vi "OP500ZP_SCANequipements.vi"(8 "Errin":errorcluster caption="errin", 10 "Chaîne":string="Log et conf\\Config.ini", 11 "pathin":path=path "D:/CODE/02 SLIM ZEN") -> (0 "ERROUT":errorcluster caption="error out", 1 "KO?":bool=TRUE, 3 "VISA OUT":T1)   [LabVIEW 2020]
doc: "Ce vi il détecte la presence des équipements"
uses:
  VG/VG_ATEQ.vi
  VG/VG_ST5520.vi
  VG/VG_BT3562.vi
  VG/VG_MX5060.vi
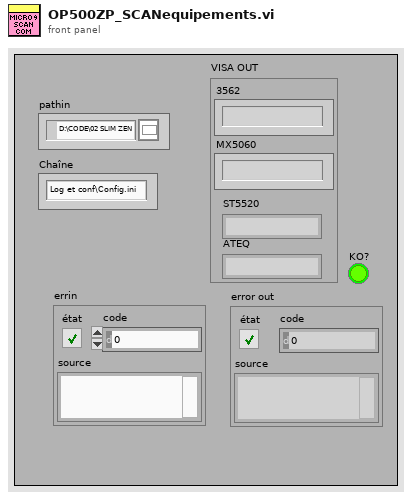
[diagram p1: front panel]
types:
  T1 = cluster{"3562":string, "MX5060":string, "ST5520":string, "ATEQ":string}
  T2 = cluster{"3564":string, "MX5060":string, "ST5520":string, "ATEQ":string}
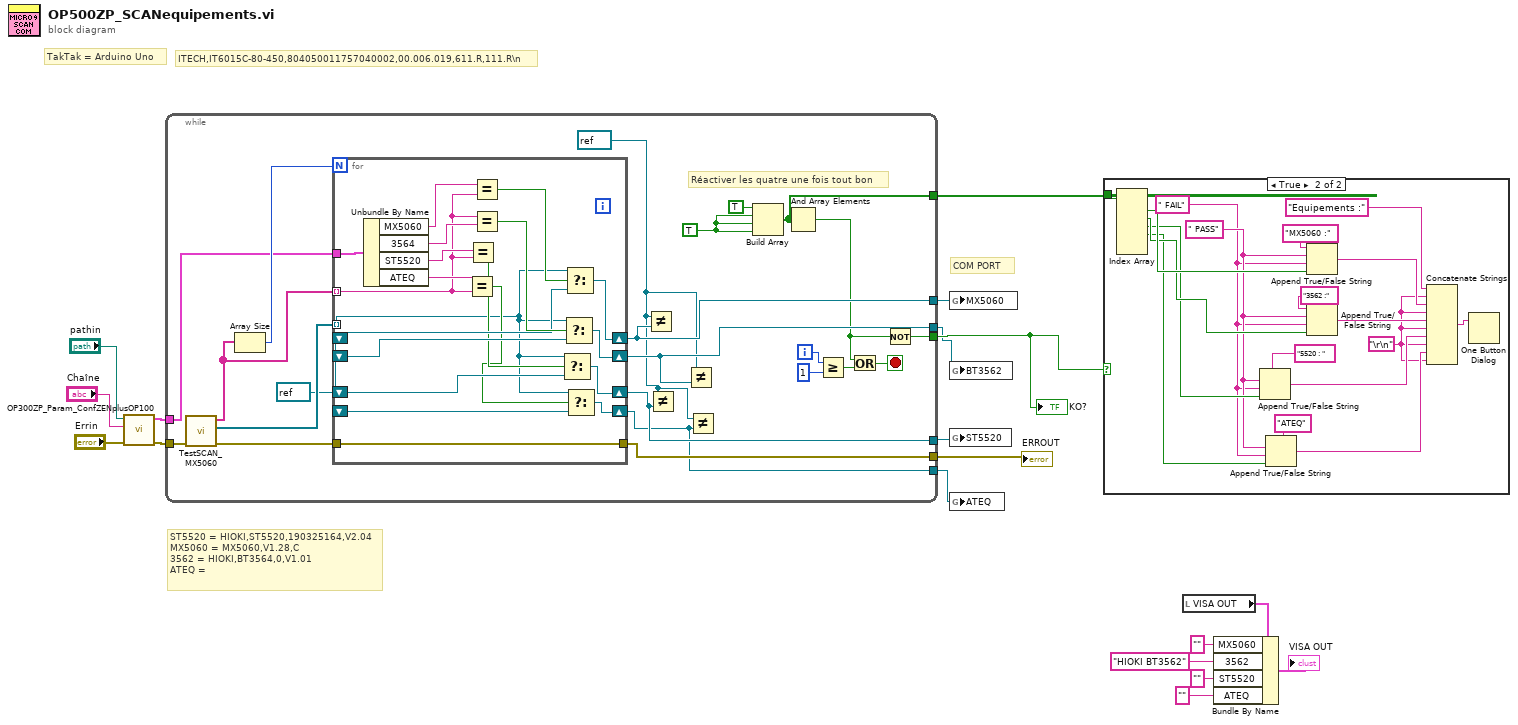
[diagram p0: block diagram]
diagram:
  # "ST5520 = HIOKI,ST5520,190325164,V2.04\t\nMX5060 = MX5060,V1.28,C\n3562 = HIOKI,BT3564,0,V1.01\nATEQ ="
  # "COM PORT"
  # "TakTak = Arduino Uno"
  # "ITECH,IT6015C-80-450,804050011757040002,00.006.019,611.R,111.R\\n"
  n1 = call "OP300ZP_Param_ConfZENplusOP100.vi"("errin"="Errin", "Chaîne"="Chaîne", "pathin"="pathin") -> ("errout"=w15:errorcluster, "VISA OUT"=w14:T2)  [unwired: 7 in]
  n2 = while {
    tunnel: [w30] -> w6
    tunnel: [w29] -> w7
    tunnel: w15 -> [w39]
    tunnel: [w34] -> w18
    tunnel: w14 -> [w31]
    tunnel: [w27] -> w17
    tunnel: [w25] -> w5
    tunnel: [w23] -> w1
    tunnel: [w21] -> w4
    i -> [w33]
    stop <- w36 stop-if-true
    w19 = TRUE ("élément")
    w22 = refnum<visa-resource-name> refnum ("x")
    w26 = refnum<visa-resource-name> refnum ("VISA resource name out")
    # "Réactiver les quatre une fois tout bon"
    n3 = call "TestSCAN_MX5060.vi"("errin"=w39) -> ("error out"=w24:errorcluster, "Tableau 2"=w37:refnum<visa-resource-name>[], "Tableau"=w38:string[])  [unwired: 8 in]
    n4 = Array Size(array=w38) -> (size(s)=w40:i32)
    n5 = for {
      N: w40 -> [_]
      shift-right: [w58] -> w30
      shift-left: w26 -> [w56]
      shift-right: [w57] -> w29
      shift-left: w26 -> [w55]
      tunnel: w38 -> [w45] mode=indexing
      tunnel: w31 -> [w54]
      shift-right: [w51] -> w25
      shift-left: w26 -> [w52]
      tunnel: w37 -> [w43] mode=indexing
      tunnel: w24 -> [w47]
      tunnel: [w47] -> w23
      shift-right: [w42] -> w21
      shift-left: _ -> [w41]
      n6 = Unbundle By Name(w54) -> ("MX5060"=w53:string, "3564"=w48:string, "ST5520"=w50:string, "ATEQ"=w46:string)
      n7 = Equal?(x=w46, y=w45) -> (x = y?=w44:bool)
      n8 = Equal?(x=w50, y=w45) -> (x = y?=w49:bool)
      n9 = Equal?(x=w53, y=w45) -> (x = y?=w59:bool)
      n10 = Equal?(x=w45, y=w48) -> (x = y?=w60:bool)
      n11 = Select(t=w43, s=w49, f=w52) -> (s? t:f=w51:refnum<visa-resource-name>)
      n12 = Select(t=w43, s=w60, f=w55) -> (s? t:f=w57:refnum<visa-resource-name>)
      n13 = Select(t=w43, s=w59, f=w56) -> (s? t:f=w58:refnum<visa-resource-name>)
      n14 = Select(t=w43, s=w44, f=w41) -> (s? t:f=w42:refnum<visa-resource-name>)
    }
    n15 = Not Equal?(x=w22, y=w30) -> ()  [unwired: 1 out]
    n16 = Not Equal?(x=w22, y=w25) -> ()  [unwired: 1 out]
    n17 = Not Equal?(x=w22, y=w29) -> ()  [unwired: 1 out]
    n18 = Not Equal?(x=w22, y=w21) -> ()  [unwired: 1 out]
    n19 = Build Array(TRUE ("élément"), w19, w19, w19) -> (w27:bool[])
    n20 = And Array Elements(Boolean array=w27) -> (logical AND=w28:bool)
    n21 = Greater Or Equal?(x=w33, y=1) -> (x >= y?=w35:bool)
    n22 = Or(x=w28, y=w35) -> (x .or. y?=w36:bool)
    n23 = Not(x=w28) -> (.not. x?=w34:bool)
  }
  "KO?" <- w18
  "ERROUT" <- w1
  n24 = global write "VG_MX5060.vi" "MX5060"(w6) -> ()
  n25 = global write "VG_BT3562.vi" "BT3562"(w7) -> ()
  n26 = global write "VG_ST5520.vi" "ST5520"(w5) -> ()
  n27 = global write "VG_ATEQ.vi" "ATEQ"(w4) -> ()
  n28 = case shown="True" w18 {
    tunnel: w17 -> [_ w70]
    frame False {
    }
    frame True {
      w61 = "\r\n"
      w65 = " PASS" ("chaîne faux")
      w64 = " FAIL" ("chaîne faux")
      n29 = Index Array(array=w70) -> (element #1=w69:bool, element #2=w68:bool, element #3=w67:bool, element #4=w63:bool)  [unwired: 6 in, 2 out]
      n30 = Append True/False String(1:w67, 2:w64, 3:w65, 4:"5520 : " ("chaîne (\"\")")) -> (0:w72:string)
      n31 = Append True/False String(1:w63, 2:w64, 3:w65, 4:"ATEQ" ("chaîne (\"\")")) -> (0:w62:string)
      n32 = Append True/False String(1:w69, 2:w64, 3:w65, 4:"MX5060 :" ("chaîne (\"\")")) -> (0:w74:string)
      n33 = Append True/False String(1:w68, 2:w64, 3:w65, 4:"3562 :" ("chaîne (\"\")")) -> (0:w73:string)
      n34 = Concatenate Strings("Equipements :" ("chaîne"), w61, w74, w61, w73, w61, w72, w61, w62, w61) -> (w71:string)
      n35 = One Button Dialog(message=w71) -> ()  [unwired: 1 in, 1 out]
    }
  }
  n36 = local read "VISA OUT"() -> (w10:T1)
  n37 = Bundle By Name(cluster=w10, "MX5060"="", "3562"="HIOKI BT3562", "ST5520"="", "ATEQ"="") -> (→"VISA OUT":T1)
